vi "temp state machine.vi"() -> ()   [LabVIEW 2012]
panel:
  in  "Thermometer":dbl(slide) scale=0.0..100.0
  out "HIGH":bool
  out "MEDIUM":bool
  out "LOW":bool
  out "Enum":enum16{"High", "Medium", "low"}(ring)
  in  "stop":bool
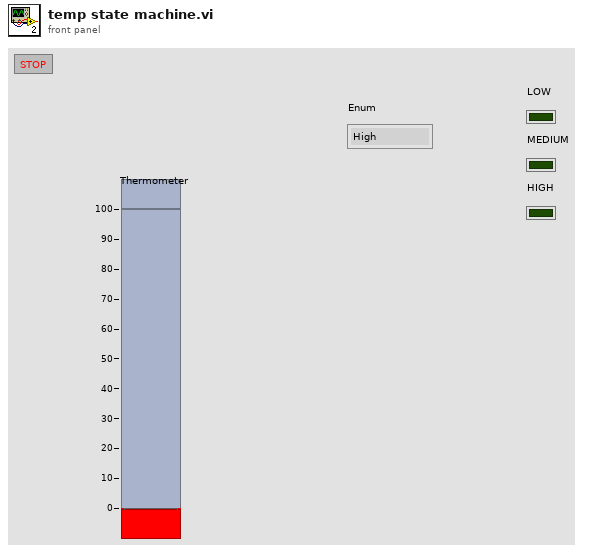
[diagram p1: front panel]
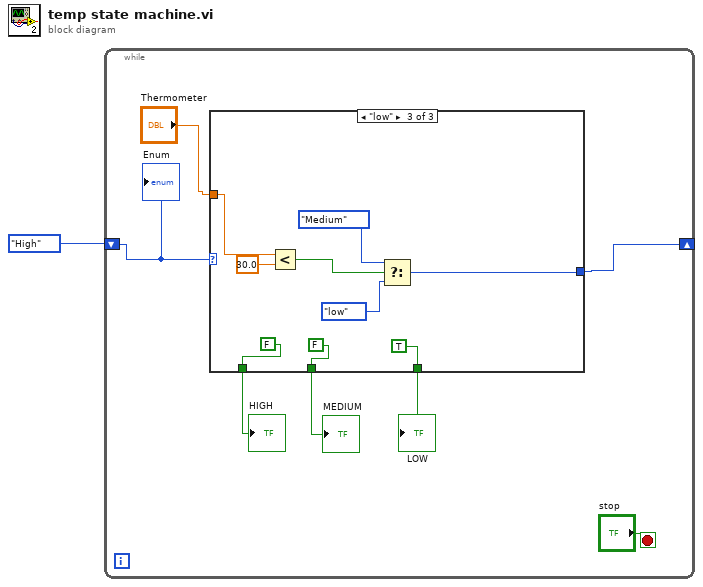
[diagram p0: block diagram]
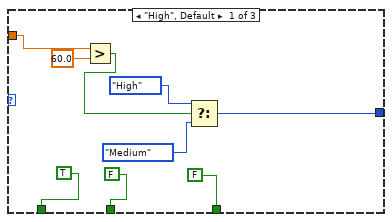
[diagram p2: hidden frame]
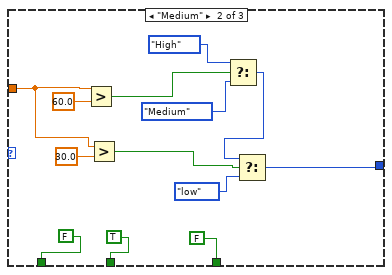
[diagram p3: hidden frame]
diagram:
  n1 = while {
    shift-right: [w2] -> _
    shift-left: enum16{"High", "Medium", "low"}."High" ("Enum") -> [w7]
    stop <- "stop" stop-if-true
    n2 = case shown="\"low\"" w7 {
      tunnel: [w15 w18 w37] -> w2
      tunnel: "Thermometer" -> [w13 w23 w36]
      tunnel: [TRUE ("HIGH") FALSE ("HIGH") FALSE ("HIGH")] -> w5
      tunnel: [FALSE ("HIGH") TRUE ("HIGH") FALSE ("HIGH")] -> w4
      tunnel: [FALSE ("HIGH") FALSE ("HIGH") TRUE ("HIGH")] -> w3
      frame "High", Default {
        n3 = Greater?(x=w13, y=60.0) -> (0:w12:bool)
        n4 = Select(t=enum16{"High", "Medium", "low"}."High" ("Enum"), s=w12, f=enum16{"High", "Medium", "low"}."Medium" ("Enum")) -> (s? t:f=w15:enum16{"High", "Medium", "low"})
      }
      frame "Medium" {
        n5 = Greater?(x=w23, y=60.0) -> (0:w22:bool)
        n6 = Greater?(x=w23, y=30.0) -> (0:w21:bool)
        n7 = Select(t=enum16{"High", "Medium", "low"}."High" ("Enum"), s=w22, f=enum16{"High", "Medium", "low"}."Medium" ("Enum")) -> (s? t:f=w19:enum16{"High", "Medium", "low"})
        n8 = Select(t=w19, s=w21, f=enum16{"High", "Medium", "low"}."low" ("Enum")) -> (s? t:f=w18:enum16{"High", "Medium", "low"})
      }
      frame "low" {
        n9 = Less?(x=w36, y=30.0) -> (x < y?=w34:bool)
        n10 = Select(t=enum16{"High", "Medium", "low"}."Medium" ("Enum"), s=w34, f=enum16{"High", "Medium", "low"}."low" ("Enum")) -> (s? t:f=w37:enum16{"High", "Medium", "low"})
      }
    }
    "LOW" <- w3
    "MEDIUM" <- w4
    "HIGH" <- w5
    "Enum" <- w7
  }
